vi "Send OCP.vi"(8 "error in (no error)":errorcluster, 11 "79XRP in":refnum<class "79XRP.lvclass">) -> (0 "error out":errorcluster, 3 "79XRP out":refnum<class "79XRP.lvclass">)   [LabVIEW 2019, in "79XRP.lvlib" / "79XRP.lvclass"]
uses:
  Library/79XRP.lvclass
  C:/Users/Public/Documents/Development/builds/Instruments/PowerSupply.lvlibp/Library/PowerSupply.lvclass
  Accessors/Read Local Resource.vi
  Accessors/Write Local Resource.vi
  <instrlib>/Keysight RP7900 Series/Keysight RP7900 Series.lvlib
  builds/Engine/Engine.lvlibp/Project/Engine.lvclass
  C:/Users/Public/Documents/Development/builds/Engine/Engine.lvlibp/Project/Engine.lvclass
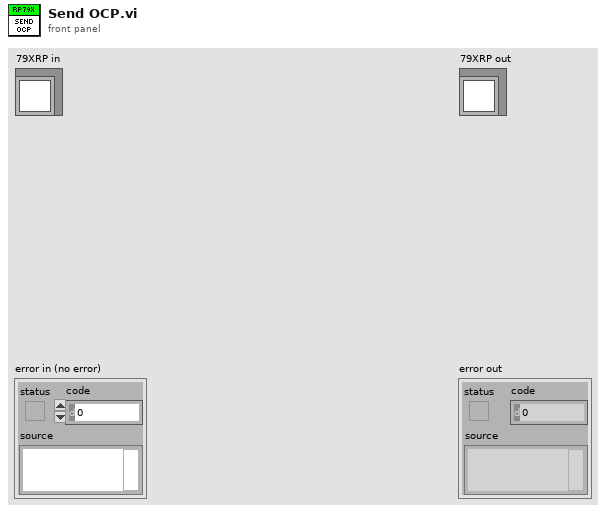
[diagram p1: front panel]
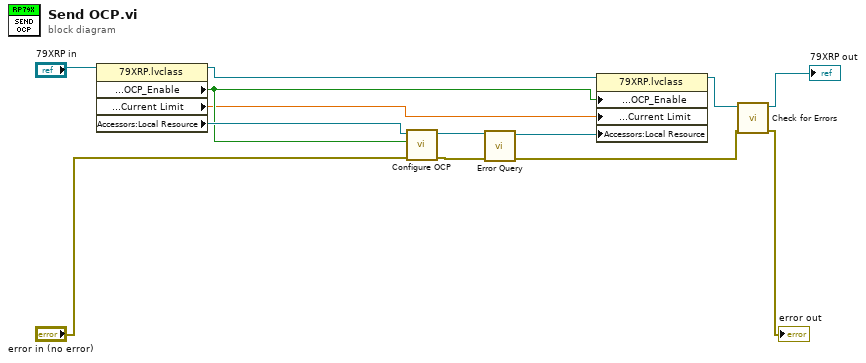
[diagram p0: block diagram]
diagram:
  n1 = property class="79XRP.lvclass"(reference="79XRP in") -> (reference out=w8:refnum<class "79XRP.lvclass">, "Accessors:Setting:Protection:OCP_Enable"=w10:bool, "Accessors:Setting:Protection:Current Limit"=w9:dbl, "Accessors:Local Resource"=w12:refnum<visa-resource-name>)  [unwired: 1 in, 1 out]
  n2 = call <instrlib>:"Configure OCP.vi"("error in (no error)"="error in (no error)", "Enable OCP (F: Disable)"=w10, "VISA resource name"=w12) -> ("error out"=w6:errorcluster, "VISA resource name out"=w7:refnum<visa-resource-name>)  [unwired: 7 in]
  n3 = call <instrlib>:"Error Query.vi"("error in (no error)"=w6, "VISA resource name"=w7) -> ("error out"=w5:errorcluster, "VISA resource name out"=w3:refnum<visa-resource-name>)  [unwired: 6 in, 2 out]
  n4 = property class="79XRP.lvclass"(reference=w8, "Accessors:Setting:Protection:OCP_Enable"=w10, "Accessors:Setting:Protection:Current Limit"=w9, "Accessors:Local Resource"=w3) -> (reference out=w2:refnum<class "79XRP.lvclass">)  [unwired: 1 in, 1 out]
  n5 = call "Check for Errors.vi"("error in"=w5, "Engine in"=w2) -> ("error out"=→"error out":errorcluster, "Engine out"=→"79XRP out":refnum<class "79XRP.lvclass">)  [unwired: 8 in]
